vi "Get Period.vi"(3 "WavBuf":refnum<class "WavBuf.lvclass">) -> (1 "Dt Out":dbl)   [LabVIEW 2024, in "WavBuf.lvclass"]
uses:
  WavBuf.lvclass
  WavBuf.lvclass/WavBuf.ctl
panel:
  out "t0":timestamp
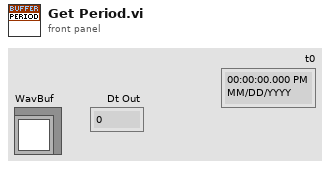
[diagram p1: front panel]
types:
  T1 = typedef "Ref_DVR_Buffer.ctl" = refnum<data-value>
  T2 = typedef "Waveform_Data.ctl" = waveform(dbl)
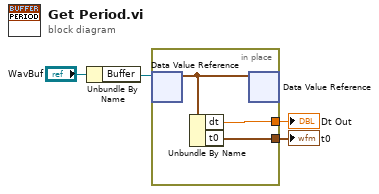
[diagram p0: block diagram]
diagram:
  n1 = Unbundle By Name("WavBuf") -> ("Buffer"=w3:T1)
  n2 = in-place {
    in-place-border: [w6] -> w2
    in-place-border: [w5] -> w1
    n3 = in-place-dvr #1(w3) -> (w7:T2)  [unwired: 1 out]
    n4 = Unbundle By Name(w7) -> ("dt"=w6:dbl, "t0"=w5:timestamp)
    n5 = in-place-dvr #1(w7) -> ()  [unwired: 2 out]
  }
  "Dt Out" <- w2
  "t0" <- w1
